vi "Configure Multi Group.vi"(0 "VISA resource name":refnum<visa-resource-name>, 1 "Batch Group Number  [/BT] (1)":i32=1 min=1 max=12, 2 "Group Number (1)":i32=1 min=1 max=12 step=1, 3 "Enable Group (False)":bool, 4 "Group Name (\"\")":string, 5 "error in (no error)":errorcluster, 7 "Channel (no array)":string[](array[string])) -> (14 "VISA resource name out":refnum<visa-resource-name>, 15 "Batch Group Number":i32, 16 "Group Number":i32, 19 "error out":errorcluster)   [LabVIEW 2020, in "Yokogawa GX Series.lvlib"]
doc: "Sets the group (/BT Option).\n\nCommand: SMltGroup"
uses:
  <instrlib>/Yokogawa GX Series/Yokogawa GX Series.lvlib
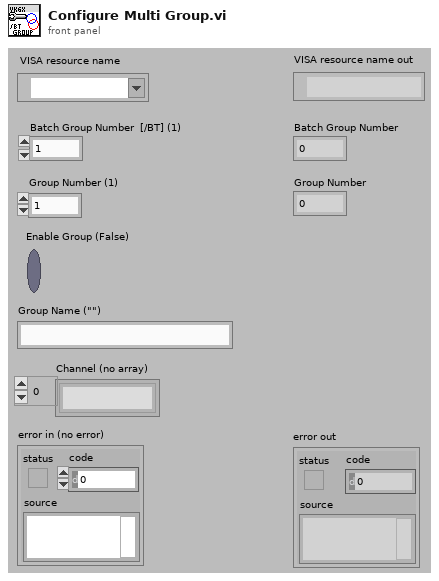
[diagram p1: front panel]
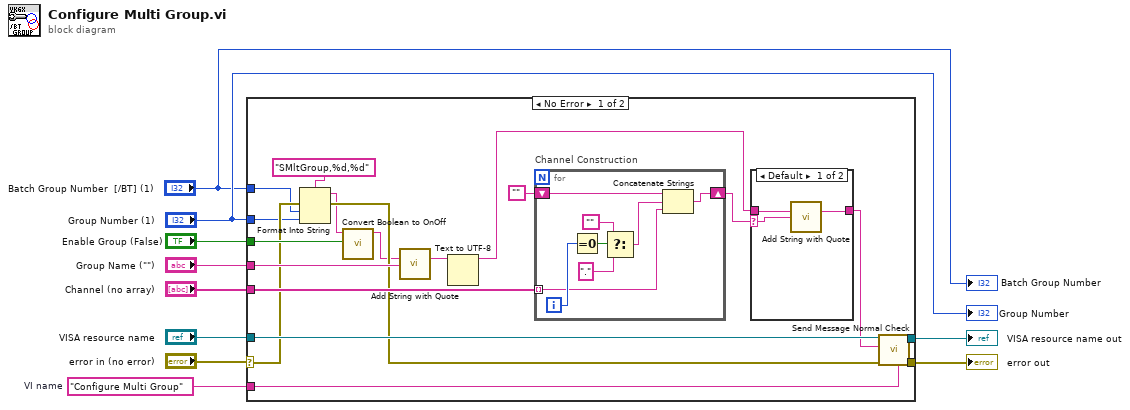
[diagram p0: block diagram]
diagram:
  w9 = "Configure Multi Group"  # VI name
  n1 = case shown="No Error" "error in (no error)" {
    selector: "error in (no error)" -> [w15 w42]
    tunnel: "Channel (no array)" -> [w28 _]
    tunnel: w9 -> [w27 _]
    tunnel: [w26 w43] -> w8
    tunnel: [w25 w42] -> w7
    tunnel: "VISA resource name" -> [w24 w43]
    tunnel: "Group Name (\"\")" -> [w23 _]
    tunnel: "Enable Group (False)" -> [w19 _]
    tunnel: "Group Number (1)" -> [w12 _]
    tunnel: "Batch Group Number  [/BT] (1)" -> [w11 _]
    frame No Error {
      n2 = Format Into String(format string="SMltGroup,%d,%d", error in=w15, w11, w12) -> (resulting string=w20:string, error out=w21:errorcluster)  [unwired: 1 in]
      n3 = call <instrlib>:"Convert Boolean to OnOff.vi"("On/Off"=w19, "Initial String (\"\")"=w20) -> ("Resulting String"=w18:string)  [unwired: 9 in]
      n4 = call <instrlib>:"Add String with Quote.vi"("Initial String (\"\")"=w18, "String (\"\")"=w23) -> ("Resulting String"=w14:string)  [unwired: 12 in, 1 out]
      n5 = Text to UTF-8(11:w14) -> (3:w13:string)  [unwired: 2 in, 1 out]
      n6 = for "Channel Construction" {
        tunnel: w28 -> [w34] mode=indexing
        shift-right: [w40] -> w17
        shift-left: "" -> [w41]
        i -> [w39]
        n7 = Equal To 0?(x=w39) -> (x = 0?=w38:bool)
        n8 = Select(t="", s=w38, f=".") -> (s? t:f=w37:string)
        n9 = Concatenate Strings(w41, w37, w34) -> (w40:string)
      }
      n10 = case shown="Default" w17 {
        selector: w17 -> [w32 _]
        tunnel: [w31 w33] -> w16
        tunnel: w13 -> [w30 w33]
        frame Default {
          n11 = call <instrlib>:"Add String with Quote.vi"("Initial String (\"\")"=w30, "String (\"\")"=w32) -> ("Resulting String"=w31:string)  [unwired: 12 in, 1 out]
        }
        frame "" {
        }
      }
      n12 = call <instrlib>:"Send Message Normal Check.vi"("Source (\"\")"=w27, "error in (no error)"=w21, "Send Message (\"\")"=w16, "VISA resource name"=w24) -> ("error out"=w25:errorcluster, "VISA resource name out"=w26:refnum<visa-resource-name>)  [unwired: 2 in, 4 out]
    }
    frame Error {
    }
  }
  "error out" <- w7
  "VISA resource name out" <- w8
  "Group Number" <- "Group Number (1)"
  "Batch Group Number" <- "Batch Group Number  [/BT] (1)"
